vi "CreateTheory.vi"(5 "Theory In":refnum<class "Theory.lvclass">, 8 "error in (no error)":errorcluster, 9 "Control Data":map{string, variant}(c390), 10 "VI Refnum":refnum<vi>) -> (0 "error out":errorcluster, 3 "Theory":refnum<class "Theory.lvclass">)   [LabVIEW 2019, in "TestCase.lvlib" / "Theory.lvclass"]
uses:
  Theory.lvclass
  C:/Users/de200256/Code/LVUnit/TestCase/Fact/Fact.lvclass
  Theory.lvclass/Theory.ctl
  Fact/Fact.lvclass
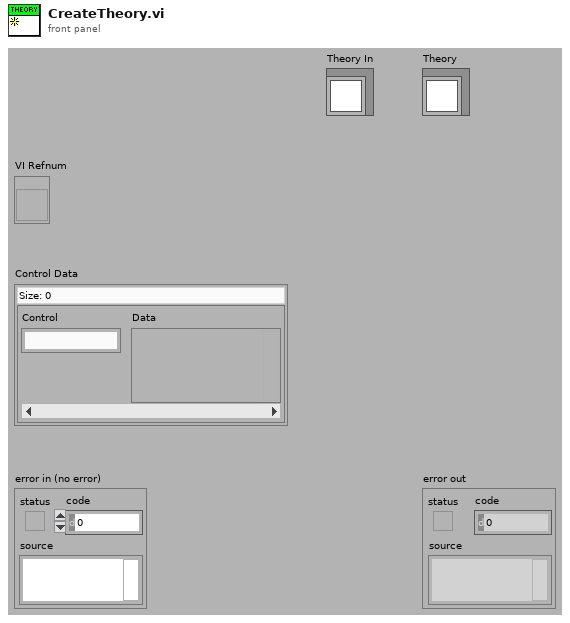
[diagram p1: front panel]
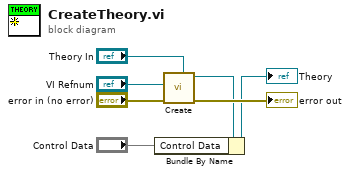
[diagram p0: block diagram]
diagram:
  n1 = call "Create.vi"("Fact In"="Theory In", "error in (no error)"="error in (no error)", "VI Refnum"="VI Refnum") -> ("error out"=→"error out":errorcluster, "Fact"=w4:refnum<class "Theory.lvclass">)  [unwired: 7 in]
  n2 = Bundle By Name(cluster=w4, "Control Data"="Control Data") -> (→"Theory":refnum<class "Theory.lvclass">)
